vi "HRM-Stage3-init_main.vi"() -> (0 "error out":errorcluster, 3 "Init cluster":T1)   [LabVIEW 2020]
uses:
  HRM-Stage3-init_cluster.ctl
  HRM-Stage3-User_events.ctl
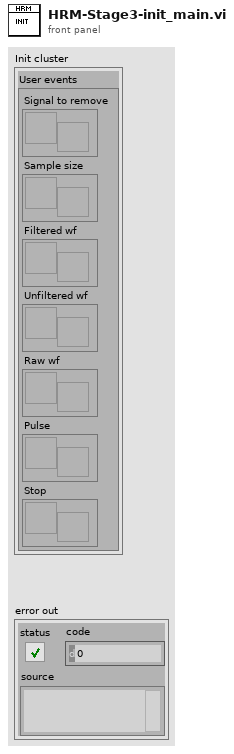
[diagram p1: front panel]
types:
  T1 = typedef "HRM-Stage3-init_cluster.ctl" = cluster{"User events":T2}
  T2 = typedef "HRM-Stage3-User_events.ctl" = cluster{"Signal to remove":refnum<user-event>, "Sample size":refnum<user-event>, "Filtered wf":refnum<user-event>, "Unfiltered wf":refnum<user-event>, "Raw wf":refnum<user-event>, "Pulse":refnum<user-event>, "Stop":refnum<user-event>}
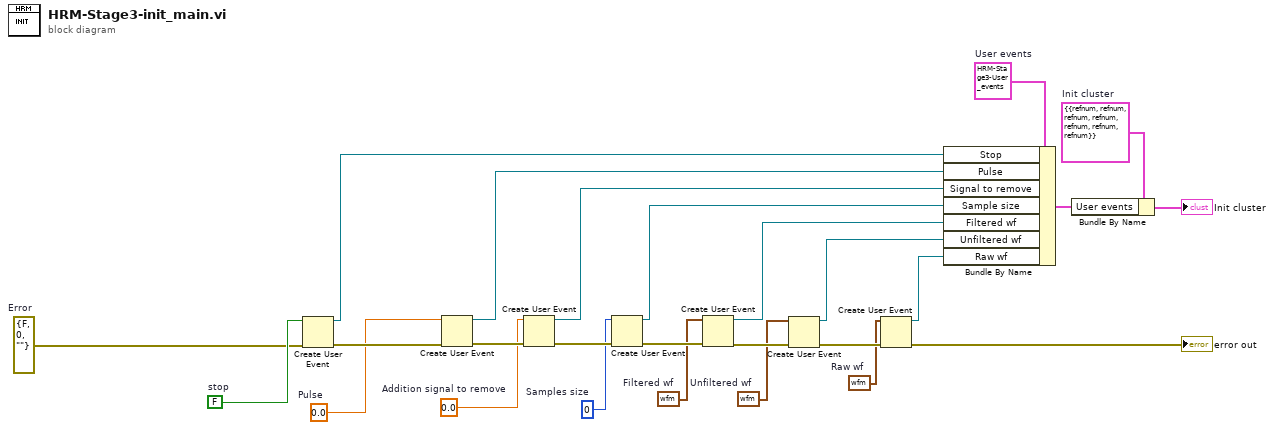
[diagram p0: block diagram]
diagram:
  w1 = errorcluster {"status"=FALSE, "code"=0, "source"=""}  # Error
  w22 = FALSE  # stop
  w20 = T1 {"User events"={"Signal to remove"=refnum, "Sample size"=refnum, "Filtered wf"=refnum, "Unfiltered wf"=refnum, "Raw wf"=refnum, "Pulse"=refnum, "Stop"=refnum}}  # Init cluster
  w17 = 0.0  # Pulse
  w11 = T2 {"Signal to remove"=refnum, "Sample size"=refnum, "Filtered wf"=refnum, "Unfiltered wf"=refnum, "Raw wf"=refnum, "Pulse"=refnum, "Stop"=refnum}  # User events
  w6 = 0  # Samples size
  w5 = 0.0  # Addition signal to remove
  w4 = waveform(dbl) {"t0"=timestamp(0 s since 1904-01-01), "dt"=1.0, "Y"=[]}  # Filtered wf
  w3 = waveform(dbl) {"t0"=timestamp(0 s since 1904-01-01), "dt"=1.0, "Y"=[]}  # Unfiltered wf
  w2 = waveform(dbl) {"t0"=timestamp(0 s since 1904-01-01), "dt"=1.0, "Y"=[]}  # Raw wf
  n1 = Create User Event(user event datatype=w22, error in=w1) -> (user event=w24:refnum<user-event>, error out=w23:errorcluster)
  n2 = Create User Event(user event datatype=w17, error in=w23) -> (user event=w18:refnum<user-event>, error out=w19:errorcluster)
  n3 = Create User Event(user event datatype=w5, error in=w19) -> (user event=w12:refnum<user-event>, error out=w10:errorcluster)
  n4 = Create User Event(user event datatype=w6, error in=w10) -> (user event=w13:refnum<user-event>, error out=w9:errorcluster)
  n5 = Create User Event(user event datatype=w4, error in=w9) -> (user event=w14:refnum<user-event>, error out=w8:errorcluster)
  n6 = Create User Event(user event datatype=w3, error in=w8) -> (user event=w15:refnum<user-event>, error out=w7:errorcluster)
  n7 = Create User Event(user event datatype=w2, error in=w7) -> (user event=w16:refnum<user-event>, error out=→"error out":errorcluster)
  n8 = Bundle By Name(cluster=w11, "Stop"=w24, "Pulse"=w18, "Signal to remove"=w12, "Sample size"=w13, "Filtered wf"=w14, "Unfiltered wf"=w15, "Raw wf"=w16) -> (w21:T2)
  n9 = Bundle By Name(cluster=w20, "User events"=w21) -> (→"Init cluster":T1)
